vi "calculate_max_activity13.vi"() -> ()   [LabVIEW 2025]
panel:
  out "Maximum Value":dbl
  out "Random Data":dbl(graph)
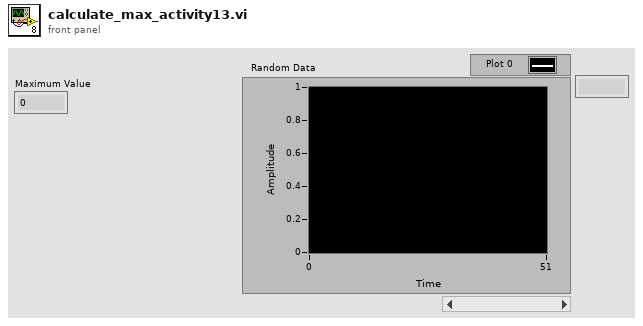
[diagram p1: front panel]
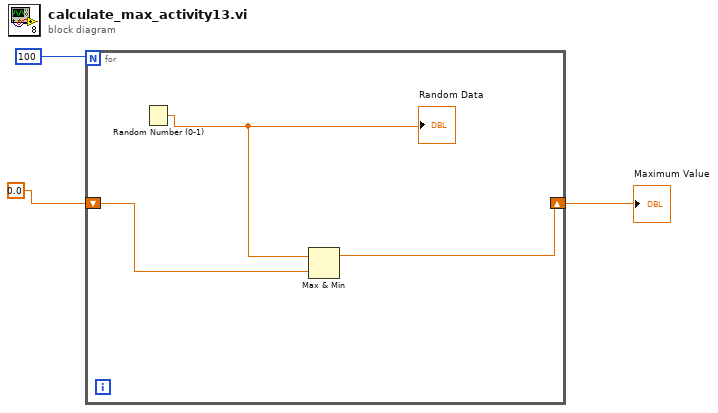
[diagram p0: block diagram]
diagram:
  n1 = for {
    N: 100 -> [_]
    shift-right: [w6] -> w1
    shift-left: 0.0 -> [w4]
    n2 = Random Number (0-1)() -> (number: 0 to 1=w5:dbl)
    "Random Data" <- w5
    n3 = Max & Min(x=w5, y=w4) -> (max(x,y)=w6:dbl)  [unwired: 1 out]
  }
  "Maximum Value" <- w1
